vi "Parse Autobuild CSV Line.vi"(3 "String":string, 5 "Autobuild root dir":path) -> (0 "Task Info":T1, 1 "Build Command":bool, 2 "Retain Build":bool)   [LabVIEW 2010]
uses:
  Types/Job Type.ctl
  Types/Task Info.ctl
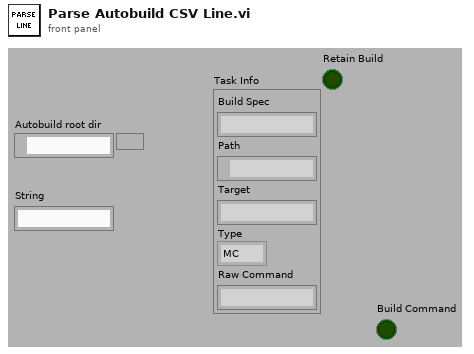
[diagram p1: front panel]
types:
  T1 = typedef "Task Info.ctl" = cluster{"Build Spec":string, "Path":path, "Target":string, "Type":T2, "Raw Command":string}
  T2 = typedef "Job Type.ctl" = enum16{"MC", "NOP", "VI", "Build", "VIP", "VIPB", "VIA"}
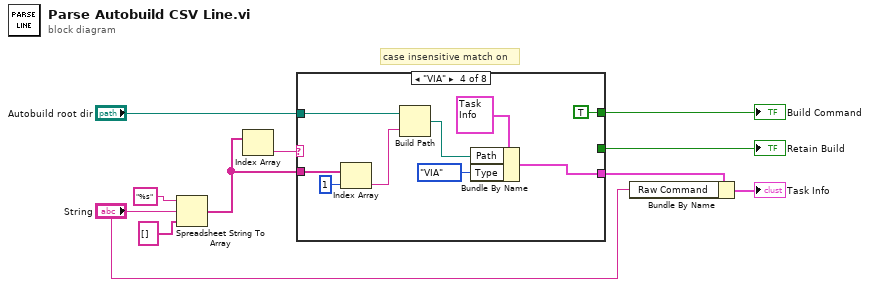
[diagram p0: block diagram]
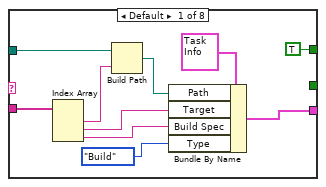
[diagram p2: hidden frame]
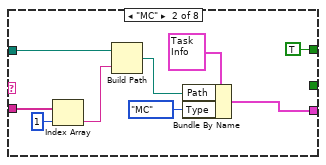
[diagram p3: hidden frame]
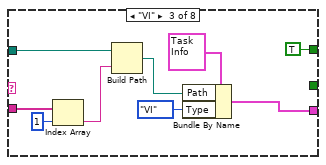
[diagram p4: hidden frame]
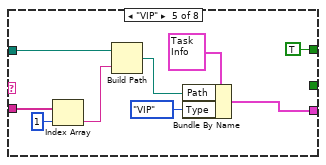
[diagram p5: hidden frame]
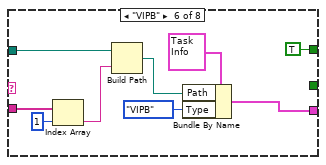
[diagram p6: hidden frame]
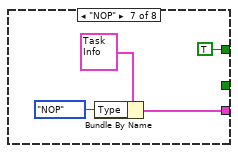
[diagram p7: hidden frame]
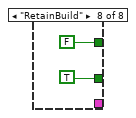
[diagram p8: hidden frame]
diagram:
  # "case insensitive match on"
  n1 = Spreadsheet String To Array(format string="%s", spreadsheet string="String", array type (2D Dbl)=string[] []) -> (array=w5:string[])  [unwired: 1 in]
  n2 = Index Array(array=w5) -> (element=w9:string)  [unwired: 1 in]
  n3 = case shown="\"VIA\"" w9 {
    tunnel: [w15 w26 w35 w44 w53 w62 w68 _] -> w10
    tunnel: w5 -> [w14 w25 w34 w43 w52 w61 _ _]
    tunnel: "Autobuild root dir" -> [w13 w24 w33 w42 w51 w60 _ _]
    tunnel: [TRUE TRUE TRUE TRUE TRUE TRUE TRUE FALSE] -> w2
    tunnel: [_ _ _ _ _ _ _ TRUE] -> w1
    frame Default {
      n4 = Index Array(array=w14) -> (element #1=w19:string, element #2=w17:string, element #3=w16:string)  [unwired: 3 in]
      n5 = Build Path(base path=w13, name or relative path=w19) -> (appended path=w18:path)
      n6 = Bundle By Name(cluster=T1 {"Build Spec"="", "Path"=path "", "Target"="My Computer", "Type"=enum."MC", "Raw Command"=""} ("Task Info"), "Path"=w18, "Target"=w17, "Build Spec"=w16, "Type"=Job_Type."Build") -> (w15:T1)
    }
    frame "MC" {
      n7 = Index Array(array=w25, index=1) -> (element=w28:string)
      n8 = Build Path(base path=w24, name or relative path=w28) -> (appended path=w27:path)
      n9 = Bundle By Name(cluster=T1 {"Build Spec"="", "Path"=path "", "Target"="My Computer", "Type"=enum."MC", "Raw Command"=""} ("Task Info"), "Path"=w27, "Type"=Job_Type."MC") -> (w26:T1)
    }
    frame "VI" {
      n10 = Index Array(array=w34, index=1) -> (element=w37:string)
      n11 = Build Path(base path=w33, name or relative path=w37) -> (appended path=w36:path)
      n12 = Bundle By Name(cluster=T1 {"Build Spec"="", "Path"=path "", "Target"="My Computer", "Type"=enum."MC", "Raw Command"=""} ("Task Info"), "Path"=w36, "Type"=Job_Type."VI") -> (w35:T1)
    }
    frame "VIA" {
      n13 = Index Array(array=w43, index=1) -> (element=w46:string)
      n14 = Build Path(base path=w42, name or relative path=w46) -> (appended path=w45:path)
      n15 = Bundle By Name(cluster=T1 {"Build Spec"="", "Path"=path "", "Target"="My Computer", "Type"=enum."MC", "Raw Command"=""} ("Task Info"), "Path"=w45, "Type"=Job_Type."VIA") -> (w44:T1)
    }
    frame "VIP" {
      n16 = Index Array(array=w52, index=1) -> (element=w55:string)
      n17 = Build Path(base path=w51, name or relative path=w55) -> (appended path=w54:path)
      n18 = Bundle By Name(cluster=T1 {"Build Spec"="", "Path"=path "", "Target"="My Computer", "Type"=enum."MC", "Raw Command"=""} ("Task Info"), "Path"=w54, "Type"=Job_Type."VIP") -> (w53:T1)
    }
    frame "VIPB" {
      n19 = Index Array(array=w61, index=1) -> (element=w64:string)
      n20 = Build Path(base path=w60, name or relative path=w64) -> (appended path=w63:path)
      n21 = Bundle By Name(cluster=T1 {"Build Spec"="", "Path"=path "", "Target"="My Computer", "Type"=enum."MC", "Raw Command"=""} ("Task Info"), "Path"=w63, "Type"=Job_Type."VIPB") -> (w62:T1)
    }
    frame "NOP" {
      n22 = Bundle By Name(cluster=T1 {"Build Spec"="", "Path"=path "", "Target"="My Computer", "Type"=enum."MC", "Raw Command"=""} ("Task Info"), "Type"=Job_Type."NOP") -> (w68:T1)
    }
    frame "RetainBuild" {
    }
  }
  "Build Command" <- w2
  "Retain Build" <- w1
  n23 = Bundle By Name(cluster=w10, "Raw Command"="String") -> (→"Task Info":T1)
